vi "Delete Compound DVR.vi"(8 "error in (no error)":errorcluster, 11 "Compound DVR in":refnum<data-value>) -> (0 "error out":errorcluster, 3 "Compound out":refnum<class "Compound.lvclass">)   [LabVIEW 2015, in "MDSplus.lvlib" / "Compound.lvclass"]
uses:
  <vilib>/MDSplus/Classes/Data_Class/Compound_Class/Compound.lvclass
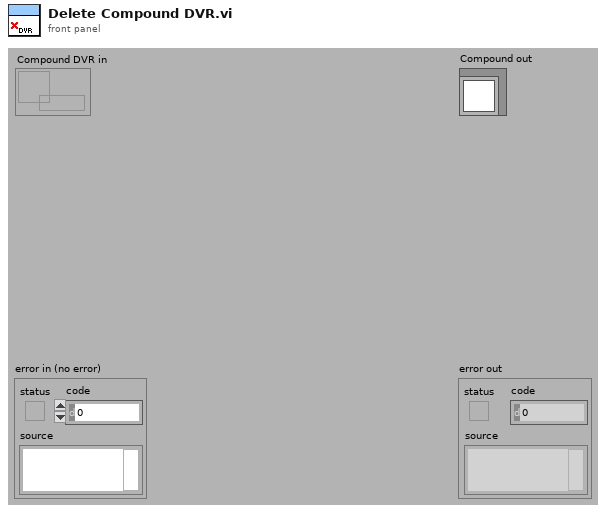
[diagram p1: front panel]
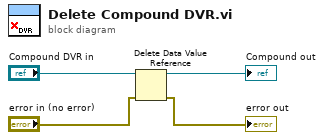
[diagram p0: block diagram]
diagram:
  n1 = Delete Data Value Reference(data value reference="Compound DVR in", error in="error in (no error)") -> (data value=→"Compound out":refnum<class "Compound.lvclass">, error out=→"error out":errorcluster)
